vi "Autonomous Independent.vi"   [LabVIEW 2014]
doc: "This VI is called when autonomous begins, and will automatically be terminated when autonomous ends. You can carry out timed or sensor driven robot movement independently without needing to return to the caller."
uses:
  <vilib>/Rock Robotics/WPI/SafetyOutput/WPI_SafetyOutputConfigMenu.ctl
  <vilib>/Rock Robotics/WPI/Solenoid/WPI_SolenoidValue.ctl
  <vilib>/Rock Robotics/WPI/Joystick/WPI_JoystickGetSetRefNum.vi
  <vilib>/Rock Robotics/Network Tables/SD Write Numeric Array.vi
  <vilib>/Rock Robotics/WPI/RobotDrive/WPI_RobotDriveGetSetRefNum.vi
  <vilib>/Rock Robotics/Network Tables/SD Read String.vi
  Robot Global Data.vi
  <vilib>/Rock Robotics/WPI/RobotDrive/WPI_RobotDriveMecanumDrive_Cartesian.vi
  <vilib>/Rock Robotics/WPI/Solenoid/WPI_SolenoidSetEnum.vi
  navx-mxp_NEW/roborio/labview/navX-MXP Library/navX-MXP IMU.lvlib
panel:
  # "EDITED: 3/2/15"
  # "Be sure to right-click and choose Data Operations>>Make Current Value default if you want to save the array values with the VI"
types:
  T1 = typedef "WPI_SafetyOutputConfigMenu.ctl" = enum16{"Enable", "Disable"}
  T2 = typedef "WPI_JoystickDevRef.ctl" = cluster{"Device":T3}
  T3 = typedef "WPI_JoystickDeviceEnum.ctl" = enum16{"USB 0", "USB 1", "USB 2", "USB 3", "USB 4", "USB 5"}
  T4 = cluster{"proportional gain (Kc)":dbl, "integral time (Ti, min)":dbl, "derivative time (Td, min)":dbl}
  T5 = typedef "WPI_RobotDriveDevRef.ctl" = cluster{"DevStatus":errorcluster, "Motors[]":T6[], "Square Inputs":bool, "Max Output":dbl}
  T6 = typedef "WPI_MotorControlDeviceRef.ctl" = cluster{"DeviceStatus":errorcluster, "Type":T7, "PWM":cluster{"Controller":T8, "PWM Channel":T9, "DeadBand":T10}, "CAN":cluster{"Device Number":u8, "Control Mode":T11, "Semaphore":T12, "Max Vout":dbl, "TalonSRX Control Mode":T13}, "Invert":bool, "TransformRef":T14, "InvTransformRef":T14}
  T7 = typedef "WPI_MotorControlType.ctl" = enum16{"PWM", "CAN", "CANTalonSRX"}
  T8 = typedef "FPGA_TypedefDigitalModule.ctl" = enum16{"Controller 1"}
  T9 = typedef "FPGA_DIOPWMChannel.ctl" = enum8{"PWM 0", "PWM 1", "PWM 2", "PWM 3", "PWM 4", "PWM 5", "PWM 6", "PWM 7", "PWM 8", "PWM 9", "PWM MXP 0", "PWM MXP 1", "PWM MXP 2", "PWM MXP 3", "PWM MXP 4", "PWM MXP 5", "PWM MXP 6", "PWM MXP 7", "PWM MXP 8", "PWM MXP 9", "Invalid"}
  T10 = typedef "WPI_PWMDeadband.ctl" = cluster{"Name":string, "maxPositivePwm":i32, "minPositivePwm":i32, "centerPwm":i32, "maxNegativePwm":i32, "minNegativePwm":i32, "angularRange":u16}
  T11 = typedef "WPI_CANJaguar_ControlMode.ctl" = enum8{"Percent VBus", "Current", "Speed", "Position", "Voltage"}
  T12 = typedef "Semaphore RefNum" = refnum<k1>
  T13 = typedef "WPI_CANTalonSRX_APIControlMode.ctl" = enum8{"Percent VBus", "Speed", "Position", "Slave", "Unchanged / Invalid"}
  T14 = typedef "WPI_PWMTransform_ConPane.ctl" = refnum<vi>
  T15 = typedef "WPI_SolenoidDevRef.ctl" = cluster{"DevStatus":errorcluster, "Pneumatics Control Module":u8, "Forward Solenoid Channel":T16, "Reverse Solenoid Channel":T16}
  T16 = typedef "WPI_SolenoidChannel.ctl" = enum8{"Solenoid 0", "Solenoid 1", "Solenoid 2", "Solenoid 3", "Solenoid 4", "Solenoid 5", "Solenoid 6", "Solenoid 7", "Invalid"}
  T17 = typedef "navX-MXP IMU.lvlib/navX Device TypeDef.ctl" = cluster{"navX Interface Protocol":T18, "navX Interface Protocol TypeDefs":cluster{"SPIDevRef":T19, "I2CDevRef":T21}, "navX System Information":cluster{"Board Information":T23, "Status":T24, "Offsets":T28}, "navX Common Information":cluster{"Update Rate (4Hz-60Hz)":T29, "refnum name":string, "error":errorcluster}}
  T18 = typedef "navX-MXP IMU.lvlib/navX Interface Protocol.ctl" = enum16{"SPI", "I2C"}
  T19 = typedef "WPI_SPIDevRef.ctl" = cluster{"DevStatus":errorcluster, "Handle":i32, "Controller":T8, "SPI Bus":T20}
  T20 = typedef "spi_bus.ctl" = enum16{"SPI On-Board, CS0", "SPI On-Board, CS1", "SPI On-Board, CS2", "SPI On-Board, CS3", "SPI MXP", "Invalid"}
  T21 = typedef "WPI_I2CDevRef.ctl" = cluster{"DevStatus":errorcluster, "Controller":T8, "Device Address":u8, "Handle":i32, "I2C Bus":T22}
  T22 = typedef "i2c_bus.ctl" = enum16{"I2C On-Board", "I2C MXP", "Invalid"}
  T23 = typedef "navX-MXP IMU.lvlib/navX Board Information.ctl" = cluster{"WhoAmI (50 | 0x32)":u8, "Board Revision":u8, "Firmware Major Version":u8, "Firmware Minor Version":u8}
  T24 = typedef "navX-MXP IMU.lvlib/navX Status Data.ctl" = cluster{"Update Rate Hz":u8, "Accelerometer Full-Scale Range":u8, "Gyro Full-Scale Range":u16, "NAVX_OP_STATUS":T25, "NAVX_CAL_STATUS":T26, "NAVX_SELFTEST_STATUS":u8, "NAVX_SENSOR_STATUS":T27}
  T25 = typedef "navX-MXP IMU.lvlib/navX NAVX_OP_STATUS.ctl" = u8
  T26 = typedef "navX-MXP IMU.lvlib/navX NAVX_CAL_STATUS.ctl" = u8
  T27 = typedef "navX-MXP IMU.lvlib/navX NAVX_SENSOR_STATUS.ctl" = cluster{"MOVING":bool, "YAW_STABLE":bool, "MAG_DISTURBANCE":bool, "ALTITUDE_VALID":bool, "SEALEVEL_PRESS_SET":bool, "FUSED_HEADING_VALID":bool}
  T28 = typedef "navX-MXP IMU.lvlib/navX Offsets Data.ctl" = cluster{"Yaw":dbl, "Quat W":dbl, "Quat X":dbl, "Quat Y":dbl, "Quat Z":dbl}
  T29 = typedef "navX-MXP IMU.lvlib/navX Update Rate.ctl" = u8
  T30 = typedef "WPI_SolenoidValue.ctl" = enum16{"Off", "On", "Forward", "Reverse"}
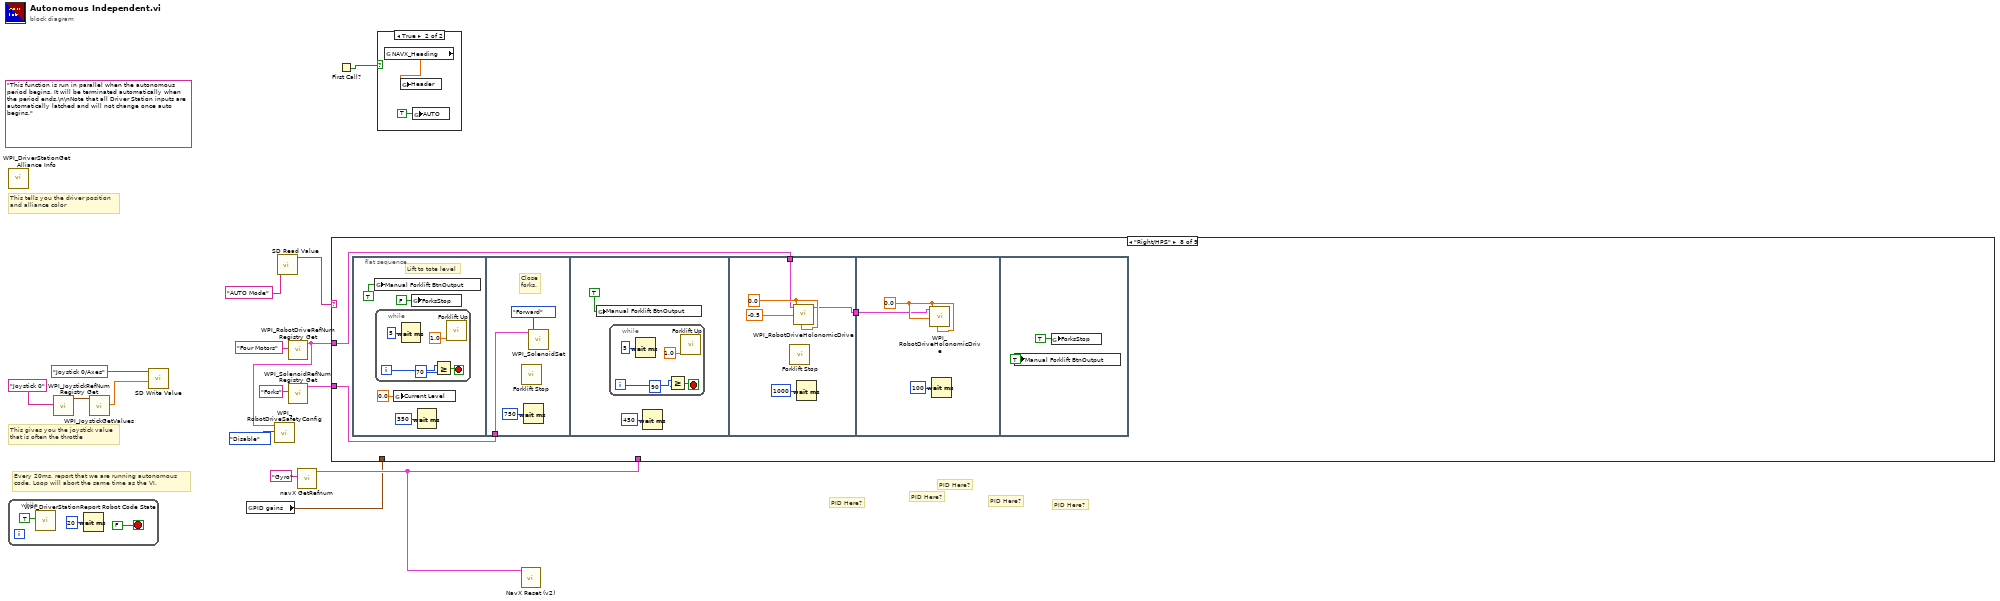
[diagram p0: block diagram]
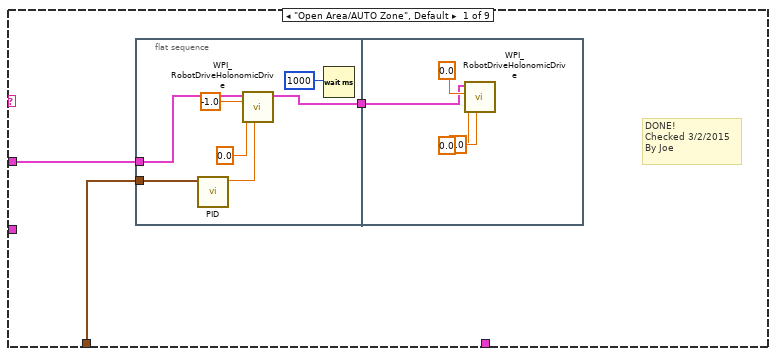
[diagram p3: hidden frame]
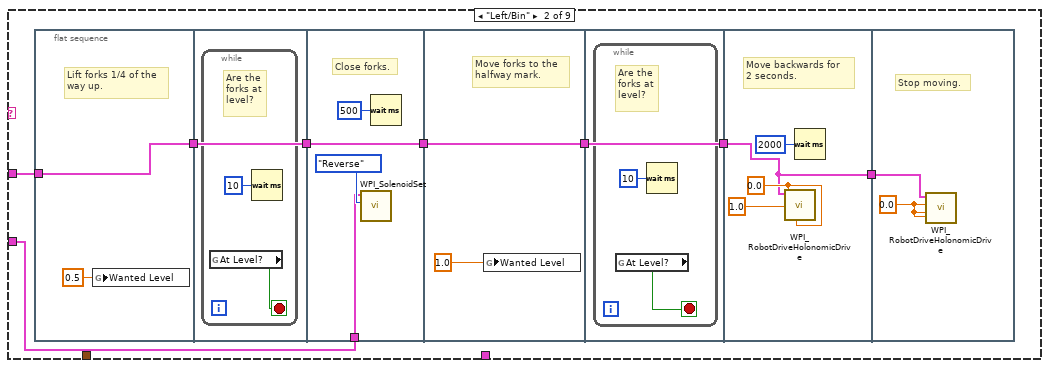
[diagram p4: hidden frame]
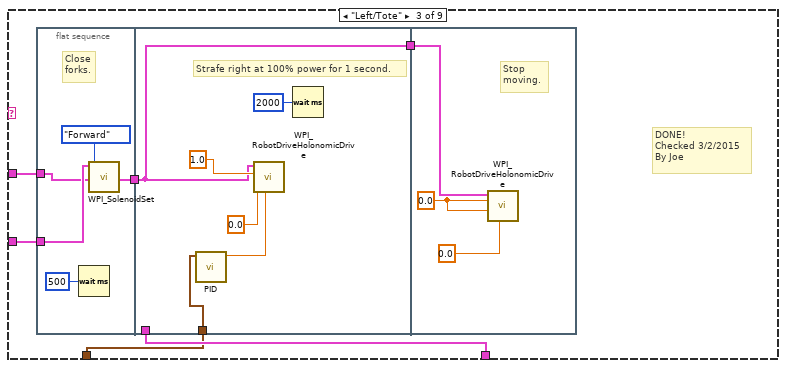
[diagram p5: hidden frame]
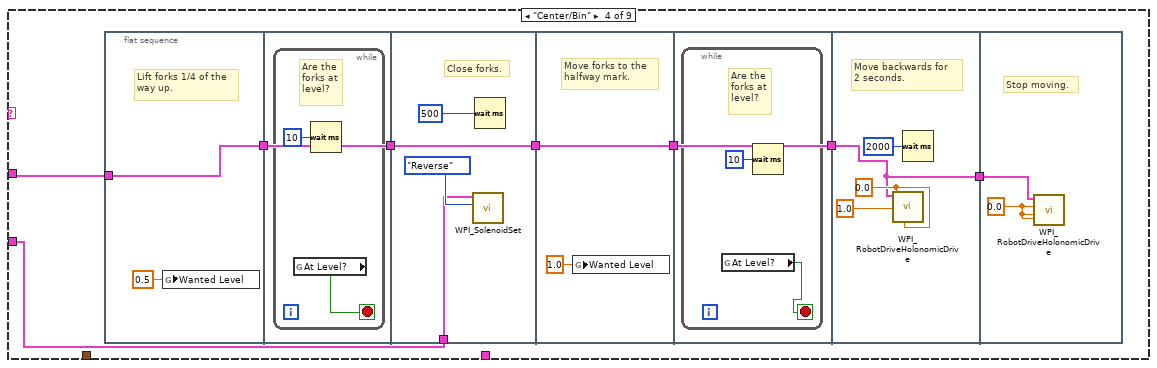
[diagram p6: hidden frame]
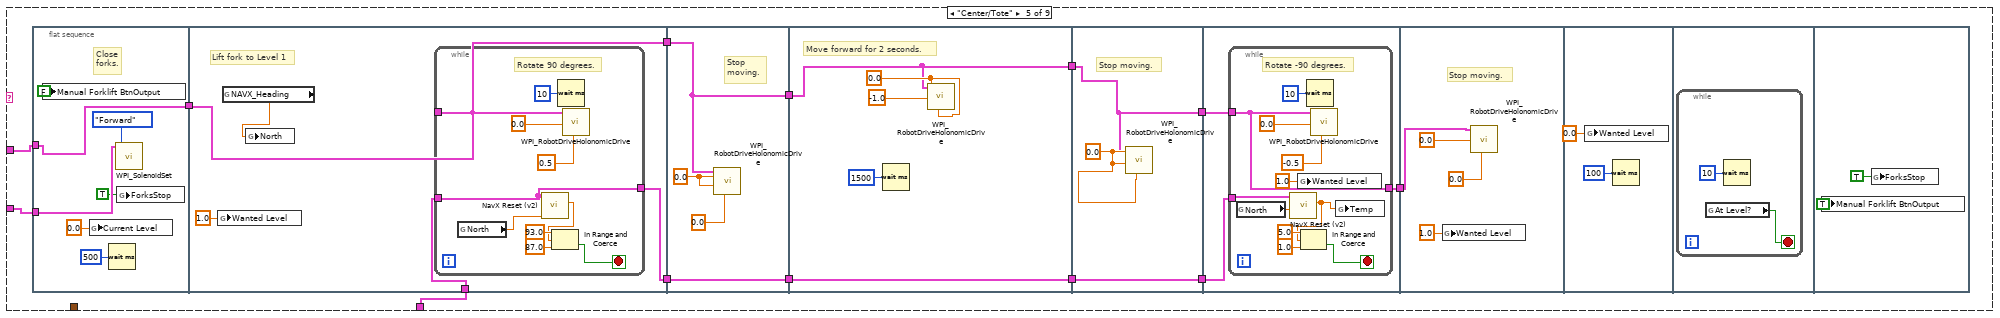
[diagram p7: hidden frame]
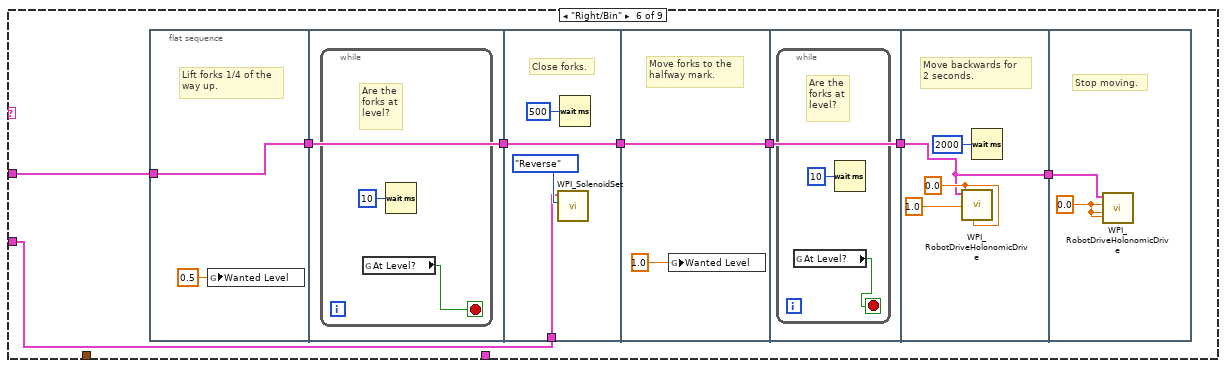
[diagram p8: hidden frame]
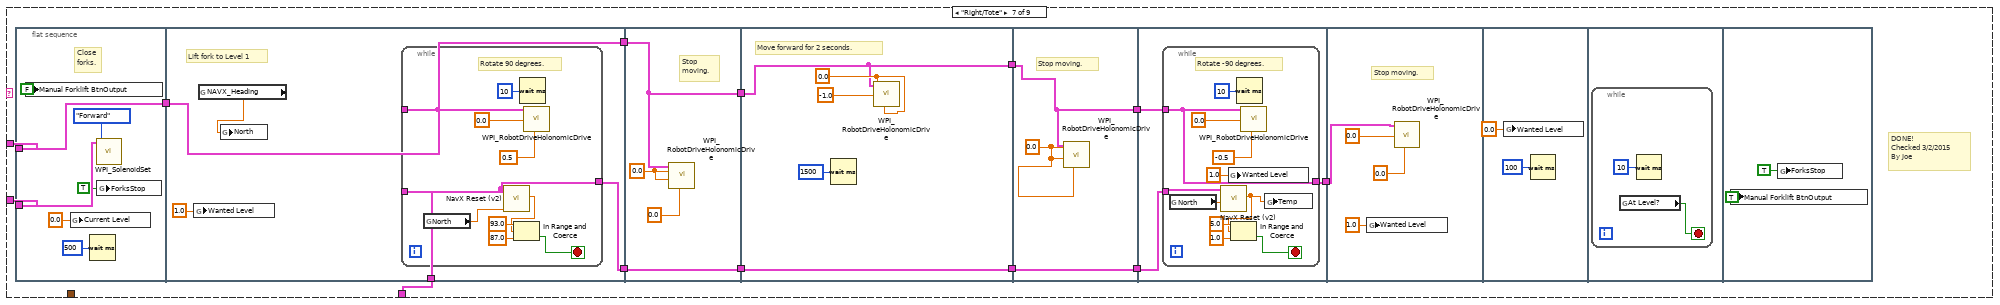
[diagram p9: hidden frame]
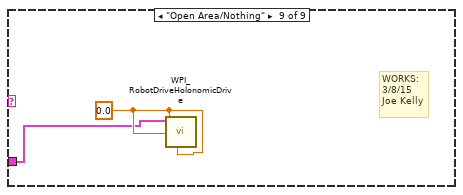
[diagram p10: hidden frame]
diagram:
  (unwired) "This function is run in parallel when the autonomous period begins. It will be terminated automatically when the period ends.\n\nNote that all Driver Station inputs are automatically latched and will not change once auto begins."
  # "PID Here?"
  # "PID Here?"
  # "PID Here?"
  # "PID Here?"
  # "PID Here?"
  # "Every 20ms, report that we are running autonomous\ncode. Loop will abort the same time as the VI."
  # "This gives you the joystick value\nthat is often the throttle"
  # "This tells you the driver position\nand alliance color"
  n1 = while {
    stop <- FALSE stop-if-true
    n2 = call <vilib>:"WPI_DriverStationReport Robot Code State.vi"("Autonomous"=TRUE) -> ()  [unwired: 10 in, 1 out]
    n3 = Wait (ms)(milliseconds to wait=u32 20) -> ()  [unwired: 1 out]
  }
  n4 = call <vilib>:"WPI_DriverStationGet Alliance Info.vi"() -> ()  [unwired: 12 out]
  n5 = call <vilib>:"WPI_JoystickRefNum Registry Get.vi"("refnum name"="Joystick 0") -> ("JoystickDevRef"=w14:T2)  [unwired: 1 in, 9 out]
  n6 = call <vilib>:"WPI_JoystickGetValues.vi"("JoystickDevRef"=w14) -> ("Axes"=w12:dbl[])  [unwired: 6 in, 4 out]
  n7 = call-poly <vilib>:"SD Write Value.vi"("Numeric Array"=w12, "Name"="Joystick 0/Axes") -> ()  [unwired: 8 in, 2 out]
  n8 = global read "Robot Global Data.vi" "PID gains"() -> (w3:T4)
  n9 = call-poly <vilib>:"SD Read Value.vi"("Name"="AUTO Mode") -> ("String"=w11:string)  [unwired: 8 in, 2 out]
  n10 = call <vilib>:"WPI_RobotDriveRefNum Registry Get.vi"("refnum name"="Four Motors") -> ("RobotDriveDevRef"=w7:T5)  [unwired: 9 in, 1 out]
  n11 = call <vilib>:"WPI_RobotDriveSafetyConfig.vi"("mode"=WPI_SafetyOutputConfigMenu."Disable", "RobotDriveDevRef"=w7) -> ()  [unwired: 8 in, 2 out]
  n12 = call <vilib>:"WPI_SolenoidRefNum Registry Get.vi"("refnum name"="Forks") -> ("SolenoidDevRef"=w8:T15)  [unwired: 9 in, 1 out]
  n13 = call "navX GetRefnum.vi"("refnum name"="Gyro") -> ("navX Device TypeDef"=w4:T17)  [unwired: 9 in, 1 out]
  n14 = case shown="\"Right/HPS\"" w11 {
    tunnel: w7 -> [w21 w39 w65 w84 w110 w184 w216 w279 w310]
    tunnel: w8 -> [_ w40 w66 w85 w109 w183 w215 w280 _]
    tunnel: w4 -> [_ _ w63 _ w108 _ w213 _ _]
    tunnel: w3 -> [w19 _ w61 _ _ _ _ _ _]
    frame "Open Area/AUTO Zone", Default {
      # "DONE!\nChecked 3/2/2015\nBy Joe"
      n15 = flat-sequence {
        tunnel: w21 -> [w25]
        tunnel: [w24] -> w20
        tunnel: w19 -> [w22]
        tunnel: w20 -> [w29]
        frame #0 {
          n16 = call "PID.vi"("PID gains"=w22) -> ("output"=w23:dbl)  [unwired: 10 in]
          n17 = call-poly <vilib>:"WPI_RobotDriveHolonomicDrive.vi"("Rotation"=w23, "Y"=0.0, "X"=-1.0, "RobotDriveDevRef"=w25) -> ("RobotDriveDevRef"=w24:T5)  [unwired: 5 in, 2 out]
          n18 = Wait (ms)(milliseconds to wait=u32 1000) -> ()  [unwired: 1 out]
        }
        frame #1 {
          n19 = call-poly <vilib>:"WPI_RobotDriveHolonomicDrive.vi"("Rotation"=0.0, "Y"=0.0, "X"=0.0, "RobotDriveDevRef"=w29) -> ()  [unwired: 5 in, 3 out]
        }
      }
    }
    frame "Left/Bin" {
      n20 = flat-sequence {
        tunnel: [w41] -> w36
        tunnel: w39 -> [w41]
        tunnel: w36 -> [w43]
        tunnel: [w43] -> w35
        tunnel: w40 -> [w48]
        tunnel: [w47] -> w37
        tunnel: w35 -> [w47]
        tunnel: w37 -> [w51]
        tunnel: [w51] -> w34
        tunnel: w34 -> [w52]
        tunnel: [w52] -> w33
        tunnel: w33 -> [w55]
        tunnel: [w55] -> w38
        tunnel: w38 -> [w59]
        frame #0 {
          # "Lift forks 1/4 of the\nway up."
          n21 = global write "Robot Global Data.vi" "Wanted Level"(0.5 ("Wanted Level")) -> ()
        }
        frame #1 {
          n22 = while {
            stop <- w45 stop-if-true
            # "Are the\nforks at\nlevel?"
            n23 = global read "Robot Global Data.vi" "At Level?"() -> (w45:bool)
            n24 = Wait (ms)(milliseconds to wait=u32 10) -> ()  [unwired: 1 out]
          }
        }
        frame #2 {
          # "Close forks."
          n25 = call-poly <vilib>:"WPI_SolenoidSet.vi"("Value"=WPI_SolenoidValue."Reverse", "SolenoidDevRef"=w48) -> ()  [unwired: 8 in, 2 out]
          n26 = Wait (ms)(milliseconds to wait=u32 500) -> ()  [unwired: 1 out]
        }
        frame #3 {
          # "Move forks to the\nhalfway mark."
          n27 = global write "Robot Global Data.vi" "Wanted Level"(1.0 ("Wanted Level")) -> ()
        }
        frame #4 {
          n28 = while {
            stop <- w54 stop-if-true
            # "Are the\nforks at\nlevel?"
            n29 = global read "Robot Global Data.vi" "At Level?"() -> (w54:bool)
            n30 = Wait (ms)(milliseconds to wait=u32 10) -> ()  [unwired: 1 out]
          }
        }
        frame #5 {
          w57 = 0.0 ("X")
          # "Move backwards for\n2 seconds."
          n31 = call-poly <vilib>:"WPI_RobotDriveHolonomicDrive.vi"("Rotation"=w57, "Y"=1.0, "X"=w57, "RobotDriveDevRef"=w55) -> ()  [unwired: 5 in, 3 out]
          n32 = Wait (ms)(milliseconds to wait=u32 2000) -> ()  [unwired: 1 out]
        }
        frame #6 {
          w60 = 0.0 ("Y")
          # "Stop moving."
          n33 = call-poly <vilib>:"WPI_RobotDriveHolonomicDrive.vi"("Rotation"=w60, "Y"=w60, "X"=w60, "RobotDriveDevRef"=w59) -> ()  [unwired: 5 in, 3 out]
        }
      }
    }
    frame "Left/Tote" {
      # "DONE!\nChecked 3/2/2015\nBy Joe"
      n34 = flat-sequence {
        tunnel: w66 -> [w69]
        tunnel: w65 -> [w68]
        tunnel: [w68] -> w62
        tunnel: w62 -> [w74]
        tunnel: [w74] -> w64
        tunnel: w63 -> [_]
        tunnel: w61 -> [w72]
        tunnel: w64 -> [w77]
        frame #0 {
          # "Close\nforks."
          n35 = Wait (ms)(milliseconds to wait=u32 500) -> ()  [unwired: 1 out]
          n36 = call-poly <vilib>:"WPI_SolenoidSet.vi"("Value"=WPI_SolenoidValue."Forward", "SolenoidDevRef"=w69) -> ()  [unwired: 8 in, 2 out]
        }
        frame #1 {
          # "Strafe right at 100% power for 1 second."
          n37 = call "PID.vi"("PID gains"=w72) -> ("output"=w71:dbl)  [unwired: 10 in]
          n38 = call-poly <vilib>:"WPI_RobotDriveHolonomicDrive.vi"("Rotation"=w71, "Y"=0.0, "X"=1.0, "RobotDriveDevRef"=w74) -> ()  [unwired: 5 in, 3 out]
          n39 = Wait (ms)(milliseconds to wait=u32 2000) -> ()  [unwired: 1 out]
        }
        frame #2 {
          w78 = 0.0 ("X")
          # "Stop\nmoving."
          n40 = call-poly <vilib>:"WPI_RobotDriveHolonomicDrive.vi"("Rotation"=0.0, "Y"=w78, "X"=w78, "RobotDriveDevRef"=w77) -> ()  [unwired: 5 in, 3 out]
        }
      }
    }
    frame "Center/Bin" {
      n41 = flat-sequence {
        tunnel: [w88] -> w83
        tunnel: w84 -> [w88]
        tunnel: w83 -> [w90]
        tunnel: [w90] -> w82
        tunnel: w85 -> [w95]
        tunnel: [w94] -> w87
        tunnel: w82 -> [w94]
        tunnel: w87 -> [w98]
        tunnel: [w98] -> w81
        tunnel: w81 -> [w99]
        tunnel: [w99] -> w80
        tunnel: w80 -> [w102]
        tunnel: [w102] -> w86
        tunnel: w86 -> [w106]
        frame #0 {
          # "Lift forks 1/4 of the\nway up."
          n42 = global write "Robot Global Data.vi" "Wanted Level"(0.5 ("Wanted Level")) -> ()
        }
        frame #1 {
          n43 = while {
            stop <- w92 stop-if-true
            # "Are the\nforks at\nlevel?"
            n44 = global read "Robot Global Data.vi" "At Level?"() -> (w92:bool)
            n45 = Wait (ms)(milliseconds to wait=u32 10) -> ()  [unwired: 1 out]
          }
        }
        frame #2 {
          # "Close forks."
          n46 = call-poly <vilib>:"WPI_SolenoidSet.vi"("Value"=WPI_SolenoidValue."Reverse", "SolenoidDevRef"=w95) -> ()  [unwired: 8 in, 2 out]
          n47 = Wait (ms)(milliseconds to wait=u32 500) -> ()  [unwired: 1 out]
        }
        frame #3 {
          # "Move forks to the\nhalfway mark."
          n48 = global write "Robot Global Data.vi" "Wanted Level"(1.0 ("Wanted Level")) -> ()
        }
        frame #4 {
          n49 = while {
            stop <- w101 stop-if-true
            # "Are the\nforks at\nlevel?"
            n50 = global read "Robot Global Data.vi" "At Level?"() -> (w101:bool)
            n51 = Wait (ms)(milliseconds to wait=u32 10) -> ()  [unwired: 1 out]
          }
        }
        frame #5 {
          w104 = 0.0 ("X")
          # "Move backwards for\n2 seconds."
          n52 = call-poly <vilib>:"WPI_RobotDriveHolonomicDrive.vi"("Rotation"=w104, "Y"=1.0, "X"=w104, "RobotDriveDevRef"=w102) -> ()  [unwired: 5 in, 3 out]
          n53 = Wait (ms)(milliseconds to wait=u32 2000) -> ()  [unwired: 1 out]
        }
        frame #6 {
          w107 = 0.0 ("Y")
          # "Stop moving."
          n54 = call-poly <vilib>:"WPI_RobotDriveHolonomicDrive.vi"("Rotation"=w107, "Y"=w107, "X"=w107, "RobotDriveDevRef"=w106) -> ()  [unwired: 5 in, 3 out]
        }
      }
    }
    frame "Center/Tote" {
      n55 = flat-sequence {
        tunnel: w109 -> [w126]
        tunnel: [w121] -> w120
        tunnel: w110 -> [w121]
        tunnel: [w132] -> w119
        tunnel: w120 -> [w132]
        tunnel: w108 -> [w130]
        tunnel: [w129] -> w118
        tunnel: w119 -> [w144]
        tunnel: [w144] -> w117
        tunnel: w118 -> [w143]
        tunnel: [w143] -> w116
        tunnel: w117 -> [w148]
        tunnel: [w148] -> w115
        tunnel: w116 -> [w147]
        tunnel: [w147] -> w114
        tunnel: w115 -> [w152]
        tunnel: w114 -> [w153]
        tunnel: [w153] -> w113
        tunnel: [w152] -> w112
        tunnel: w113 -> [w157]
        tunnel: w112 -> [w156]
        tunnel: [w155] -> w111
        tunnel: w111 -> [w170]
        frame #0 {
          # "Close\nforks."
          n56 = global write "Robot Global Data.vi" "Manual Forklift BtnOutput"(FALSE ("Manual Forklift BtnOutput")) -> ()
          n57 = global write "Robot Global Data.vi" "Current Level"(0.0 ("Current Level")) -> ()
          n58 = Wait (ms)(milliseconds to wait=u32 500) -> ()  [unwired: 1 out]
          n59 = call-poly <vilib>:"WPI_SolenoidSet.vi"("Value"=WPI_SolenoidValue."Forward", "SolenoidDevRef"=w126) -> ()  [unwired: 8 in, 2 out]
          n60 = global write "Robot Global Data.vi" "ForksStop"(TRUE ("ForksStop")) -> ()
        }
        frame #1 {
          # "Lift fork to Level 1"
          n61 = global write "Robot Global Data.vi" "Wanted Level"(1.0 ("Wanted Level")) -> ()
          n62 = global read "Robot Global Data.vi" "NAVX_Heading"() -> (w128:dbl)
          n63 = global write "Robot Global Data.vi" "North"(w128) -> ()
          n64 = while {
            tunnel: w132 -> [w142]
            tunnel: w130 -> [w134]
            tunnel: [w134] -> w129
            stop <- w138 stop-if-true
            w139 = 0.0 ("X")
            # "Rotate 90 degrees."
            n65 = global read "Robot Global Data.vi" "North"() -> (w133:dbl)
            n66 = call "NavX Reset (v2).vi"("North In"=w133, "navX Device TypeDef"=w134) -> ("Output Angle"=w135:dbl)  [unwired: 9 in]
            n67 = In Range and Coerce(upper limit=93.0, x=w135, lower limit=87.0) -> (In Range?=w138:bool)  [unwired: 1 out]
            n68 = Wait (ms)(milliseconds to wait=u32 10) -> ()  [unwired: 1 out]
            n69 = call-poly <vilib>:"WPI_RobotDriveHolonomicDrive.vi"("Rotation"=0.5, "Y"=w139, "X"=w139, "RobotDriveDevRef"=w142) -> ()  [unwired: 5 in, 3 out]
          }
        }
        frame #2 {
          w145 = 0.0 ("X")
          # "Stop\nmoving."
          n70 = call-poly <vilib>:"WPI_RobotDriveHolonomicDrive.vi"("Rotation"=0.0, "Y"=w145, "X"=w145, "RobotDriveDevRef"=w144) -> ()  [unwired: 5 in, 3 out]
        }
        frame #3 {
          w150 = 0.0 ("X")
          # "Move forward for 2 seconds."
          n71 = Wait (ms)(milliseconds to wait=u32 1500) -> ()  [unwired: 1 out]
          n72 = call-poly <vilib>:"WPI_RobotDriveHolonomicDrive.vi"("Rotation"=w150, "Y"=-1.0, "X"=w150, "RobotDriveDevRef"=w148) -> ()  [unwired: 5 in, 3 out]
        }
        frame #4 {
          w154 = 0.0 ("X")
          # "Stop moving."
          n73 = call-poly <vilib>:"WPI_RobotDriveHolonomicDrive.vi"("Rotation"=w154, "Y"=w154, "X"=w154, "RobotDriveDevRef"=w152) -> ()  [unwired: 5 in, 3 out]
        }
        frame #5 {
          n74 = while {
            tunnel: w156 -> [w161]
            tunnel: w157 -> [w162]
            tunnel: [w161] -> w155
            stop <- w165 stop-if-true
            w166 = 0.0 ("X")
            # "Rotate -90 degrees."
            n75 = global read "Robot Global Data.vi" "North"() -> (w160:dbl)
            n76 = call "NavX Reset (v2).vi"("North In"=w160, "navX Device TypeDef"=w162) -> ("Output Angle"=w158:dbl)  [unwired: 9 in]
            n77 = global write "Robot Global Data.vi" "Wanted Level"(1.0 ("Wanted Level")) -> ()
            n78 = In Range and Coerce(upper limit=5.0, x=w158, lower limit=1.0) -> (In Range?=w165:bool)  [unwired: 1 out]
            n79 = Wait (ms)(milliseconds to wait=u32 10) -> ()  [unwired: 1 out]
            n80 = call-poly <vilib>:"WPI_RobotDriveHolonomicDrive.vi"("Rotation"=-0.5, "Y"=w166, "X"=w166, "RobotDriveDevRef"=w161) -> ()  [unwired: 5 in, 3 out]
            n81 = global write "Robot Global Data.vi" "Temp"(w158) -> ()
          }
        }
        frame #6 {
          w172 = 0.0 ("X")
          # "Stop moving."
          n82 = global write "Robot Global Data.vi" "Wanted Level"(1.0 ("Wanted Level")) -> ()
          n83 = call-poly <vilib>:"WPI_RobotDriveHolonomicDrive.vi"("Rotation"=0.0, "Y"=w172, "X"=w172, "RobotDriveDevRef"=w170) -> ()  [unwired: 5 in, 3 out]
        }
        frame #7 {
          n84 = global write "Robot Global Data.vi" "Wanted Level"(0.0 ("Wanted Level")) -> ()
          n85 = Wait (ms)(milliseconds to wait=u32 100) -> ()  [unwired: 1 out]
        }
        frame #8 {
          n86 = while {
            stop <- w176 stop-if-true
            n87 = global read "Robot Global Data.vi" "At Level?"() -> (w176:bool)
            n88 = Wait (ms)(milliseconds to wait=u32 10) -> ()  [unwired: 1 out]
          }
        }
        frame #9 {
          n89 = global write "Robot Global Data.vi" "Manual Forklift BtnOutput"(TRUE ("Manual Forklift BtnOutput")) -> ()
          n90 = global write "Robot Global Data.vi" "ForksStop"(TRUE ("ForksStop")) -> ()
        }
      }
    }
    frame "Right/Bin" {
      n91 = flat-sequence {
        tunnel: [w187] -> w182
        tunnel: w184 -> [w187]
        tunnel: w182 -> [w189]
        tunnel: [w189] -> w181
        tunnel: w183 -> [w194]
        tunnel: [w193] -> w186
        tunnel: w181 -> [w193]
        tunnel: w186 -> [w197]
        tunnel: [w197] -> w180
        tunnel: w180 -> [w198]
        tunnel: [w198] -> w179
        tunnel: w179 -> [w201]
        tunnel: [w201] -> w185
        tunnel: w185 -> [w205]
        frame #0 {
          # "Lift forks 1/4 of the\nway up."
          n92 = global write "Robot Global Data.vi" "Wanted Level"(0.5 ("Wanted Level")) -> ()
        }
        frame #1 {
          n93 = while {
            stop <- w190 stop-if-true
            # "Are the\nforks at\nlevel?"
            n94 = global read "Robot Global Data.vi" "At Level?"() -> (w190:bool)
            n95 = Wait (ms)(milliseconds to wait=u32 10) -> ()  [unwired: 1 out]
          }
        }
        frame #2 {
          # "Close forks."
          n96 = call-poly <vilib>:"WPI_SolenoidSet.vi"("Value"=WPI_SolenoidValue."Reverse", "SolenoidDevRef"=w194) -> ()  [unwired: 8 in, 2 out]
          n97 = Wait (ms)(milliseconds to wait=u32 500) -> ()  [unwired: 1 out]
        }
        frame #3 {
          # "Move forks to the\nhalfway mark."
          n98 = global write "Robot Global Data.vi" "Wanted Level"(1.0 ("Wanted Level")) -> ()
        }
        frame #4 {
          n99 = while {
            stop <- w200 stop-if-true
            # "Are the\nforks at\nlevel?"
            n100 = global read "Robot Global Data.vi" "At Level?"() -> (w200:bool)
            n101 = Wait (ms)(milliseconds to wait=u32 10) -> ()  [unwired: 1 out]
          }
        }
        frame #5 {
          w203 = 0.0 ("X")
          # "Move backwards for\n2 seconds."
          n102 = call-poly <vilib>:"WPI_RobotDriveHolonomicDrive.vi"("Rotation"=w203, "Y"=1.0, "X"=w203, "RobotDriveDevRef"=w201) -> ()  [unwired: 5 in, 3 out]
          n103 = Wait (ms)(milliseconds to wait=u32 2000) -> ()  [unwired: 1 out]
        }
        frame #6 {
          w206 = 0.0 ("Y")
          # "Stop moving."
          n104 = call-poly <vilib>:"WPI_RobotDriveHolonomicDrive.vi"("Rotation"=w206, "Y"=w206, "X"=w206, "RobotDriveDevRef"=w205) -> ()  [unwired: 5 in, 3 out]
        }
      }
    }
    frame "Right/Tote" {
      # "DONE!\nChecked 3/2/2015\nBy Joe"
      n105 = flat-sequence {
        tunnel: w215 -> [w225]
        tunnel: w216 -> [w224]
        tunnel: [w224] -> w219
        tunnel: [w231] -> w218
        tunnel: w219 -> [w231]
        tunnel: w213 -> [w229]
        tunnel: [w228] -> w212
        tunnel: w218 -> [w243]
        tunnel: [w243] -> w217
        tunnel: w212 -> [w242]
        tunnel: [w242] -> w211
        tunnel: w217 -> [w247]
        tunnel: [w247] -> w214
        tunnel: w211 -> [w246]
        tunnel: [w246] -> w210
        tunnel: w214 -> [w251]
        tunnel: w210 -> [w252]
        tunnel: [w252] -> w209
        tunnel: [w251] -> w208
        tunnel: w209 -> [w256]
        tunnel: w208 -> [w255]
        tunnel: [w254] -> w207
        tunnel: w207 -> [w269]
        frame #0 {
          # "Close\nforks."
          n106 = global write "Robot Global Data.vi" "Manual Forklift BtnOutput"(FALSE ("Manual Forklift BtnOutput")) -> ()
          n107 = global write "Robot Global Data.vi" "Current Level"(0.0 ("Current Level")) -> ()
          n108 = Wait (ms)(milliseconds to wait=u32 500) -> ()  [unwired: 1 out]
          n109 = call-poly <vilib>:"WPI_SolenoidSet.vi"("Value"=WPI_SolenoidValue."Forward", "SolenoidDevRef"=w225) -> ()  [unwired: 8 in, 2 out]
          n110 = global write "Robot Global Data.vi" "ForksStop"(TRUE ("ForksStop")) -> ()
        }
        frame #1 {
          # "Lift fork to Level 1"
          n111 = global write "Robot Global Data.vi" "Wanted Level"(1.0 ("Wanted Level")) -> ()
          n112 = global read "Robot Global Data.vi" "NAVX_Heading"() -> (w227:dbl)
          n113 = global write "Robot Global Data.vi" "North"(w227) -> ()
          n114 = while {
            tunnel: w231 -> [w241]
            tunnel: w229 -> [w233]
            tunnel: [w233] -> w228
            stop <- w237 stop-if-true
            w238 = 0.0 ("X")
            # "Rotate 90 degrees."
            n115 = global read "Robot Global Data.vi" "North"() -> (w232:dbl)
            n116 = call "NavX Reset (v2).vi"("North In"=w232, "navX Device TypeDef"=w233) -> ("Output Angle"=w234:dbl)  [unwired: 9 in]
            n117 = In Range and Coerce(upper limit=93.0, x=w234, lower limit=87.0) -> (In Range?=w237:bool)  [unwired: 1 out]
            n118 = Wait (ms)(milliseconds to wait=u32 10) -> ()  [unwired: 1 out]
            n119 = call-poly <vilib>:"WPI_RobotDriveHolonomicDrive.vi"("Rotation"=0.5, "Y"=w238, "X"=w238, "RobotDriveDevRef"=w241) -> ()  [unwired: 5 in, 3 out]
          }
        }
        frame #2 {
          w244 = 0.0 ("X")
          # "Stop\nmoving."
          n120 = call-poly <vilib>:"WPI_RobotDriveHolonomicDrive.vi"("Rotation"=0.0, "Y"=w244, "X"=w244, "RobotDriveDevRef"=w243) -> ()  [unwired: 5 in, 3 out]
        }
        frame #3 {
          w249 = 0.0 ("X")
          # "Move forward for 2 seconds."
          n121 = Wait (ms)(milliseconds to wait=u32 1500) -> ()  [unwired: 1 out]
          n122 = call-poly <vilib>:"WPI_RobotDriveHolonomicDrive.vi"("Rotation"=w249, "Y"=-1.0, "X"=w249, "RobotDriveDevRef"=w247) -> ()  [unwired: 5 in, 3 out]
        }
        frame #4 {
          w253 = 0.0 ("X")
          # "Stop moving."
          n123 = call-poly <vilib>:"WPI_RobotDriveHolonomicDrive.vi"("Rotation"=w253, "Y"=w253, "X"=w253, "RobotDriveDevRef"=w251) -> ()  [unwired: 5 in, 3 out]
        }
        frame #5 {
          n124 = while {
            tunnel: w255 -> [w260]
            tunnel: w256 -> [w261]
            tunnel: [w260] -> w254
            stop <- w264 stop-if-true
            w265 = 0.0 ("X")
            # "Rotate -90 degrees."
            n125 = global read "Robot Global Data.vi" "North"() -> (w259:dbl)
            n126 = call "NavX Reset (v2).vi"("North In"=w259, "navX Device TypeDef"=w261) -> ("Output Angle"=w257:dbl)  [unwired: 9 in]
            n127 = global write "Robot Global Data.vi" "Wanted Level"(1.0 ("Wanted Level")) -> ()
            n128 = In Range and Coerce(upper limit=5.0, x=w257, lower limit=1.0) -> (In Range?=w264:bool)  [unwired: 1 out]
            n129 = Wait (ms)(milliseconds to wait=u32 10) -> ()  [unwired: 1 out]
            n130 = call-poly <vilib>:"WPI_RobotDriveHolonomicDrive.vi"("Rotation"=-0.5, "Y"=w265, "X"=w265, "RobotDriveDevRef"=w260) -> ()  [unwired: 5 in, 3 out]
            n131 = global write "Robot Global Data.vi" "Temp"(w257) -> ()
          }
        }
        frame #6 {
          w271 = 0.0 ("X")
          # "Stop moving."
          n132 = global write "Robot Global Data.vi" "Wanted Level"(1.0 ("Wanted Level")) -> ()
          n133 = call-poly <vilib>:"WPI_RobotDriveHolonomicDrive.vi"("Rotation"=0.0, "Y"=w271, "X"=w271, "RobotDriveDevRef"=w269) -> ()  [unwired: 5 in, 3 out]
        }
        frame #7 {
          n134 = global write "Robot Global Data.vi" "Wanted Level"(0.0 ("Wanted Level")) -> ()
          n135 = Wait (ms)(milliseconds to wait=u32 100) -> ()  [unwired: 1 out]
        }
        frame #8 {
          n136 = while {
            stop <- w275 stop-if-true
            n137 = global read "Robot Global Data.vi" "At Level?"() -> (w275:bool)
            n138 = Wait (ms)(milliseconds to wait=u32 10) -> ()  [unwired: 1 out]
          }
        }
        frame #9 {
          n139 = global write "Robot Global Data.vi" "Manual Forklift BtnOutput"(TRUE ("Manual Forklift BtnOutput")) -> ()
          n140 = global write "Robot Global Data.vi" "ForksStop"(TRUE ("ForksStop")) -> ()
        }
      }
    }
    frame "Right/HPS" {
      n141 = flat-sequence {
        tunnel: w280 -> [w290]
        tunnel: w279 -> [w302]
        tunnel: [w300] -> w278
        tunnel: w278 -> [w306]
        frame #0 {
          # "Lift to tote level"
          n142 = global write "Robot Global Data.vi" "Manual Forklift BtnOutput"(TRUE ("Manual Forklift BtnOutput")) -> ()
          n143 = while {
            i -> [w286]
            stop <- w287 stop-if-true
            n144 = Wait (ms)(milliseconds to wait=u32 5) -> ()  [unwired: 1 out]
            n145 = Greater Or Equal?(x=w286, y=70) -> (x >= y?=w287:bool)
            n146 = call "Forklift Up.vi"("Forklift Up Power"=1.0) -> ()  [unwired: 11 in]
          }
          n147 = global write "Robot Global Data.vi" "Current Level"(0.0 ("Current Level")) -> ()
          n148 = global write "Robot Global Data.vi" "ForksStop"(FALSE ("ForksStop")) -> ()
          n149 = Wait (ms)(milliseconds to wait=u32 350) -> ()  [unwired: 1 out]
        }
        frame #1 {
          # "Close\nforks."
          n150 = call "Forklift Stop.vi"() -> ()  [unwired: 12 in]
          n151 = Wait (ms)(milliseconds to wait=u32 750) -> ()  [unwired: 1 out]
          n152 = call-poly <vilib>:"WPI_SolenoidSet.vi"("Value"=WPI_SolenoidValue."Forward", "SolenoidDevRef"=w290) -> ()  [unwired: 8 in, 2 out]
        }
        frame #2 {
          n153 = global write "Robot Global Data.vi" "Manual Forklift BtnOutput"(TRUE ("Manual Forklift BtnOutput")) -> ()
          n154 = while {
            i -> [w296]
            stop <- w297 stop-if-true
            n155 = Wait (ms)(milliseconds to wait=u32 5) -> ()  [unwired: 1 out]
            n156 = Greater Or Equal?(x=w296, y=90) -> (x >= y?=w297:bool)
            n157 = call "Forklift Up.vi"("Forklift Up Power"=1.0) -> ()  [unwired: 11 in]
          }
          n158 = Wait (ms)(milliseconds to wait=u32 450) -> ()  [unwired: 1 out]
        }
        frame #3 {
          w303 = 0.0 ("X")
          n159 = call "Forklift Stop.vi"() -> ()  [unwired: 12 in]
          n160 = call-poly <vilib>:"WPI_RobotDriveHolonomicDrive.vi"("Rotation"=w303, "Y"=-0.5, "X"=w303, "RobotDriveDevRef"=w302) -> ("RobotDriveDevRef"=w300:T5)  [unwired: 5 in, 2 out]
          n161 = Wait (ms)(milliseconds to wait=u32 1000) -> ()  [unwired: 1 out]
        }
        frame #4 {
          w307 = 0.0 ("X")
          n162 = call-poly <vilib>:"WPI_RobotDriveHolonomicDrive.vi"("Rotation"=w307, "Y"=w307, "X"=w307, "RobotDriveDevRef"=w306) -> ()  [unwired: 5 in, 3 out]
          n163 = Wait (ms)(milliseconds to wait=u32 100) -> ()  [unwired: 1 out]
        }
        frame #5 {
          n164 = global write "Robot Global Data.vi" "Manual Forklift BtnOutput"(TRUE ("Manual Forklift BtnOutput")) -> ()
          n165 = global write "Robot Global Data.vi" "ForksStop"(TRUE ("ForksStop")) -> ()
        }
      }
    }
    frame "Open Area/Nothing" {
      w311 = 0.0 ("X")
      # "WORKS:\n3/8/15\nJoe Kelly"
      n166 = call-poly <vilib>:"WPI_RobotDriveHolonomicDrive.vi"("Rotation"=w311, "Y"=w311, "X"=w311, "RobotDriveDevRef"=w310) -> ()  [unwired: 5 in, 3 out]
    }
  }
  n167 = First Call?() -> (First Call?: T/F=w1:bool)
  n168 = case shown="True" w1 {
    frame False {
    }
    frame True {
      n169 = global read "Robot Global Data.vi" "NAVX_Heading"() -> (w313:dbl)
      n170 = global write "Robot Global Data.vi" "Header"(w313) -> ()
      n171 = global write "Robot Global Data.vi" "AUTO"(TRUE ("AUTO")) -> ()
    }
  }
  n172 = call "NavX Reset (v2).vi"("navX Device TypeDef"=w4) -> ()  [unwired: 10 in, 1 out]
